vi "LHF.DB.Mongo.Collection.Core.AggregateV.vi"(6 "Extract ObjectID":bool, 7 "type":variant, 8 "error in (no error)":errorcluster, 9 "Collection":string, 10 "operations":refnum<k24>[](array[refnum]), 11 "LHF.DB.Mongo in":refnum<class "LHF.DB.Mongo.lvclass">) -> (0 "error out":errorcluster, 1 "Documents":variant[](array[variant]), 2 "operations out":refnum<k24>[](array[refnum]), 3 "LHF.DB.Mongo out":refnum<class "LHF.DB.Mongo.lvclass">, 5 "ObjectID":string[](array[string]))   [LabVIEW 2013, in "LHF.DB.Mongo.lvclass"]
uses:
  LHF.DB.Mongo.lvclass
  C:/Users/schim/Desktop/Projetos/LabVIEW-MongoDB/src/Driver/MongoDB.Bson.dll
  Driver/MongoDB.Bson.dll
  C:/Users/schim/Desktop/Projetos/LabVIEW-MongoDB/src/Driver/MongoDB.Driver.dll
  Driver/MongoDB.Driver.dll
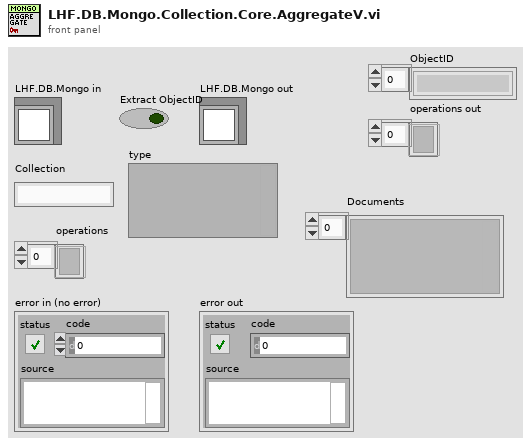
[diagram p1: front panel]
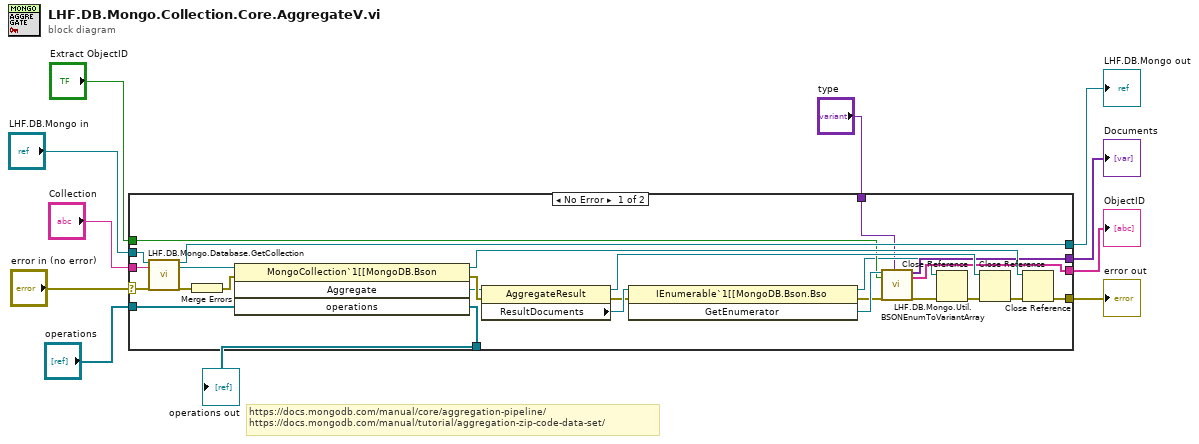
[diagram p0: block diagram]
diagram:
  # "https://docs.mongodb.com/manual/core/aggregation-pipeline/\nhttps://docs.mongodb.com/manual/tutorial/aggregation-zip-code-data-set/"
  n1 = case shown="No Error" "error in (no error)" {
    selector: "error in (no error)" -> [w19 w40]
    tunnel: "operations" -> [w37 w38]
    tunnel: "LHF.DB.Mongo in" -> [w28 w39]
    tunnel: [w27 w39] -> w9
    tunnel: "Collection" -> [w26 _]
    tunnel: [w22 _] -> w7
    tunnel: [w20 w40] -> w6
    tunnel: [w18 _] -> w4
    tunnel: "Extract ObjectID" -> [w17 _]
    tunnel: [w13 w38] -> w2
    tunnel: "type" -> [w12 _]
    frame No Error {
      n2 = call "LHF.DB.Mongo.Database.GetCollection.vi"("LHF.DB.Mongo in"=w28, "collectionName"=w26, "error in (no error)"=w19) -> ("LHF.DB.Mongo in"=w27:refnum<class "LHF.DB.Mongo.lvclass">, "MongoCollection"=w30:refnum<k24>, "error out"=w31:errorcluster)  [unwired: 14 in]
      n3 = Merge Errors(w31) -> (w32:errorcluster)
      n4 = invoke class="MongoCollection`1[[MongoDB.Bson" method="Aggregate"(reference=w30, error in=w32, "operations"=w37) -> (reference out=w36:refnum<k24>, error out=w33:errorcluster, "Aggregate"=w29:refnum<k24>, "operations"=w13:refnum<k24>[])  [unwired: 1 in]
      n5 = property class="AggregateResult"(reference=w29, error in=w33) -> (reference out=w34:refnum<k24>, error out=w21:errorcluster, "ResultDocuments"=w25:refnum<k24>)
      n6 = invoke class="IEnumerable`1[[MongoDB.Bson.Bso" method="GetEnumerator"(reference=w25, error in=w21) -> (reference out=w16:refnum<k24>, error out=w23:errorcluster, "GetEnumerator"=w24:refnum<k24>)  [unwired: 1 in]
      n7 = call "LHF.DB.Mongo.Util.BSONEnumToVariantArray.vi"("BsonENUM"=w24, "Extract ObjectID"=w17, "error in (no error)"=w23, "type"=w12) -> ("Documents"=w22:variant[], "ObjectIDs"=w18:string[], "error out"=w15:errorcluster)  [unwired: 13 in]
      n8 = Close Reference(reference=w16, error in (no error)=w15) -> (error out=w14:errorcluster)
      n9 = Close Reference(reference=w34, error in (no error)=w14) -> (error out=w35:errorcluster)
      n10 = Close Reference(reference=w36, error in (no error)=w35) -> (error out=w20:errorcluster)
    }
    frame Error {
    }
  }
  "error out" <- w6
  "Documents" <- w7
  "LHF.DB.Mongo out" <- w9
  "ObjectID" <- w4
  "operations out" <- w2
